vi "set_z_offset.vi"(4 "error in (no error)":errorcluster, 5 "Value":dbl[unit], 6 "Container State":T4, 7 "Display State In":T1={"control refs"={"z offset"=refnum, "laser intensity"=refnum, "XY graph"=refnum}, "error"={"status"=FALSE, "code"=0, "source"=""}, "free-run?"=TRUE, "settings"={"fix points"=[], "A"=0.0, "lambda"=0.0, "C"=0.0}, "range (um)"=0, "interpolate?"=FALSE}) -> (0 "error out":errorcluster, 3 "Display State Out":T1={"control refs"={"z offset"=refnum, "laser intensity"=refnum, "XY graph"=refnum}, "error"={"status"=FALSE, "code"=0, "source"=""}, "free-run?"=TRUE, "settings"={"fix points"=[], "A"=0.0, "lambda"=0.0, "C"=0.0}, "range (um)"=0, "interpolate?"=FALSE})   [LabVIEW 2010, in "XIntensityCompensation.xctl"]
uses:
  XIntensityCompensation.xctl
  <vilib>/_xctls/Container State.ctl
  state.ctl
  control_refs.ctl
  settings_cluster.ctl
  <vilib>/_xctls/XControlSupport.lvlib
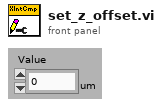
[diagram p1: front panel]
types:
  T1 = typedef "XIntensityCompensation.xctl/state.ctl" = cluster{"control refs":T2, "error":errorcluster, "free-run?":bool, "settings":T3, "range (um)":i32, "interpolate?":bool}
  T2 = typedef "XIntensityCompensation.xctl/control_refs.ctl" = cluster{"z offset":refnum<vi>, "laser intensity":refnum<vi>, "XY graph":refnum<vi>}
  T3 = typedef "XIntensityCompensation.xctl/settings_cluster.ctl" = cluster{"fix points":cluster{"depth":dbl[unit], "intensity":dbl}[], "A":dbl, "lambda":dbl[unit], "C":dbl}
  T4 = typedef "XControlSupport.lvlib/Container State.ctl" = cluster{"Indicator?":bool, "Run Mode?":bool, " Refnum":refnum<vi>}
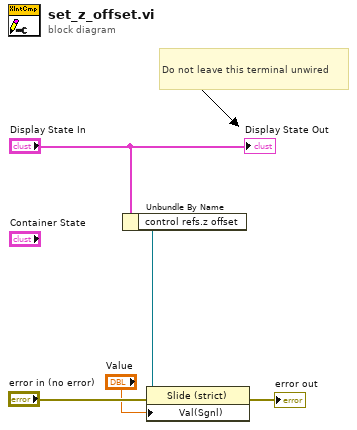
[diagram p0: block diagram]
diagram:
  # "Do not leave this terminal unwired"
  n1 = Unbundle By Name("Display State In") -> ("control refs.z offset"=w4:refnum<vi>)
  n2 = property class="Slide (strict)"(reference=w4, error in="error in (no error)", "Val(Sgnl)"="Value") -> (error out=→"error out":errorcluster)  [unwired: 1 out]
  "Display State Out" <- "Display State In"
